vi "Bool to String.vi"(1 "type (True/False)":enum16{"True/False", "on.png/off.png"}(ring), 2 "Boolean":bool) -> (0 "Bool String":string)   [LabVIEW 2016, in "Common.lvlib"]
uses:
  <userlib>/Common Components/Common/Common.lvlib
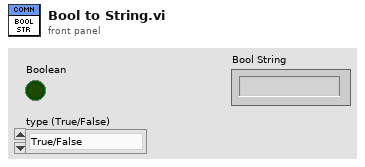
[diagram p1: front panel]
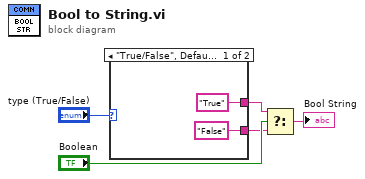
[diagram p0: block diagram]
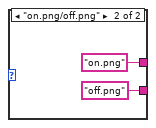
[diagram p2: hidden frame]
diagram:
  n1 = case shown="\"True/False\", Default" "type (True/False)" {
    tunnel: ["True" "on.png"] -> w4
    tunnel: ["False" "off.png"] -> w3
    frame "True/False", Default {
    }
    frame "on.png/off.png" {
    }
  }
  n2 = Select(t=w4, s="Boolean", f=w3) -> (s? t:f=→"Bool String":string)
